vi "Parse Mode.vi"(8 "error in (no error)":errorcluster, 10 "Protocol Mode in":string, 11 "File Parser Interface in":refnum<class "File Parser Interface.lvclass">) -> (0 "error out":errorcluster, 3 "File Parser Interface Out":refnum<class "File Parser Interface.lvclass">)   [LabVIEW 2018, in "File Parser Interface.lvlib" / "File Parser Interface.lvclass"]
uses:
  File Parser Interface.lvclass
  File Parser Interface.lvclass/File Parser Interface.ctl
  Read Protocol Type.vi
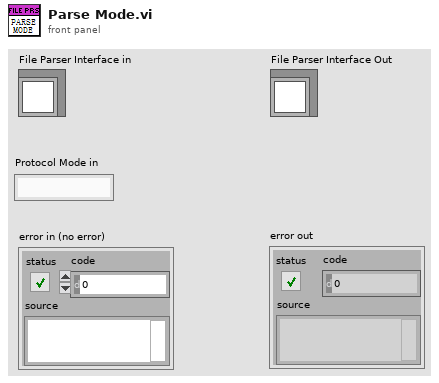
[diagram p1: front panel]
types:
  T1 = typedef "Protocol Type.ctl" = enum16{"BML_LS", "BML_HS", "SPI_3W", "SPI_4W"}
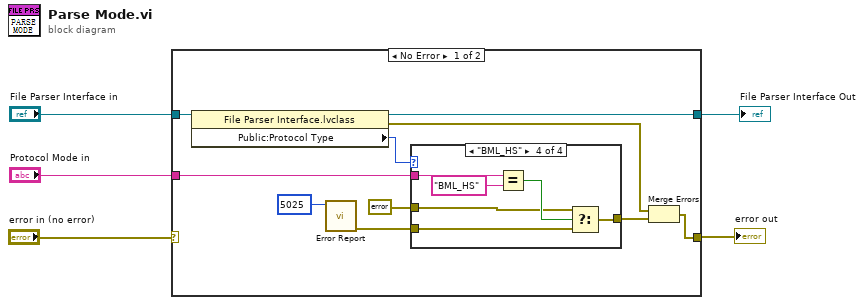
[diagram p0: block diagram]
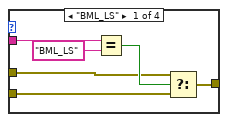
[diagram p2: hidden frame]
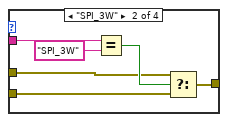
[diagram p3: hidden frame]
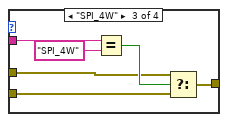
[diagram p4: hidden frame]
diagram:
  n1 = case shown="No Error" "error in (no error)" {
    selector: "error in (no error)" -> [_ w41]
    tunnel: "Protocol Mode in" -> [w12 _]
    tunnel: [w6 w41] -> w3
    tunnel: "File Parser Interface in" -> [w15 w40]
    tunnel: [w13 w40] -> w1
    frame No Error {
      n2 = property class="File Parser Interface.lvclass"(reference=w15) -> (reference out=w13:refnum<class "File Parser Interface.lvclass">, error out=w7:errorcluster, "Public:Protocol Type"=w14:T1)  [unwired: 1 in]
      n3 = call "Error Report.vi"("Error Code"=i16 5025) -> ("error out"=w10:errorcluster)  [unwired: 10 in]
      n4 = case shown="\"BML_HS\"" w14 {
        tunnel: w12 -> [w21 w27 w33 w39]
        tunnel: w10 -> [w18 w24 w30 w36]
        tunnel: errorcluster {"status"=FALSE, "code"=0, "source"=""} ("t") -> [w17 w23 w29 w35]
        tunnel: [w16 w22 w28 w34] -> w8
        frame "BML_LS" {
          n5 = Equal?(x=w21, y="BML_LS") -> (x = y?=w19:bool)
          n6 = Select(t=w17, s=w19, f=w18) -> (s? t:f=w16:errorcluster)
        }
        frame "SPI_3W" {
          n7 = Equal?(x=w27, y="SPI_3W") -> (x = y?=w25:bool)
          n8 = Select(t=w23, s=w25, f=w24) -> (s? t:f=w22:errorcluster)
        }
        frame "SPI_4W" {
          n9 = Equal?(x=w33, y="SPI_4W") -> (x = y?=w31:bool)
          n10 = Select(t=w29, s=w31, f=w30) -> (s? t:f=w28:errorcluster)
        }
        frame "BML_HS" {
          n11 = Equal?(x=w39, y="BML_HS") -> (x = y?=w37:bool)
          n12 = Select(t=w35, s=w37, f=w36) -> (s? t:f=w34:errorcluster)
        }
      }
      n13 = Merge Errors(w7, w8) -> (w6:errorcluster)
    }
    frame Error {
    }
  }
  "error out" <- w3
  "File Parser Interface Out" <- w1
